vi "Pedestal ChooseCentral.vi"() -> (1 "Central pixels":u8[](array[numeric]))   [LabVIEW 2015, in "VIPM2.lvlib"]
doc: "Opens a new window to choose how many central pixels to run."
uses:
  VIPM2.lvlib
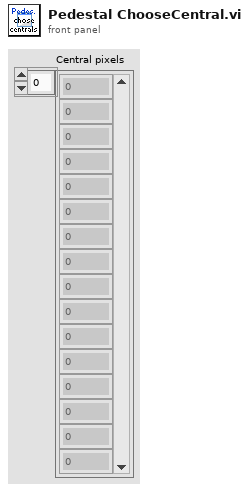
[diagram p1: front panel]
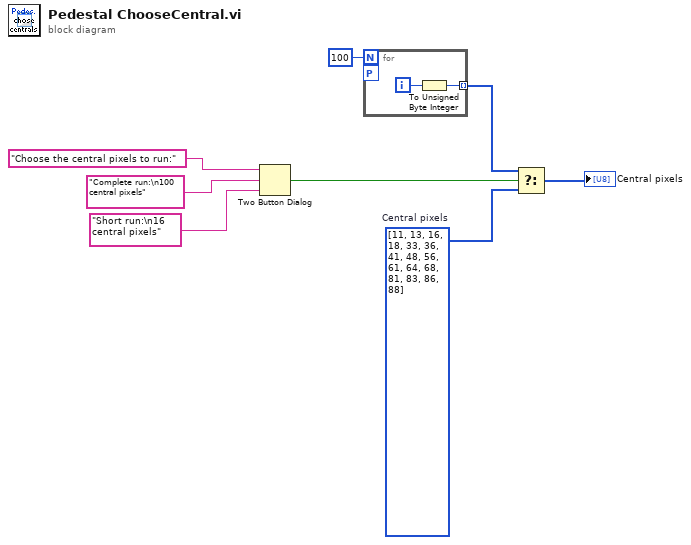
[diagram p0: block diagram]
diagram:
  w2 = u8[] [11, 13, 16, 18, 33, 36, 41, 48, 56, 61, 64, 68, 81, 83, 86, 88]  # Central pixels
  n1 = Two Button Dialog(message="Choose the central pixels to run:", 1:"Short run:\n16 central pixels" ("T button name (\"OK\")"), 2:"Complete run:\n100 central pixels" ("T button name (\"OK\")")) -> (T button?=w4:bool)
  n2 = for {
    N: 100 -> [_]
    tunnel: [w9] -> w3 mode=indexing
    workers-P: _ -> [_]
    i -> [w10]
    n3 = To Unsigned Byte Integer(number=w10) -> (unsigned 8bit integer=w9:u8)
  }
  n4 = Select(t=w3, s=w4, f=w2) -> (s? t:f=→"Central pixels":u8[])
